vi "test_assignment.vi"() -> ()   [LabVIEW 2019]
panel:
  in  "OK Button":bool
  out "Indicator":bool
  out "x+y":dbl
  in  "tempInC":dbl(knob) scale=0.0..10.0
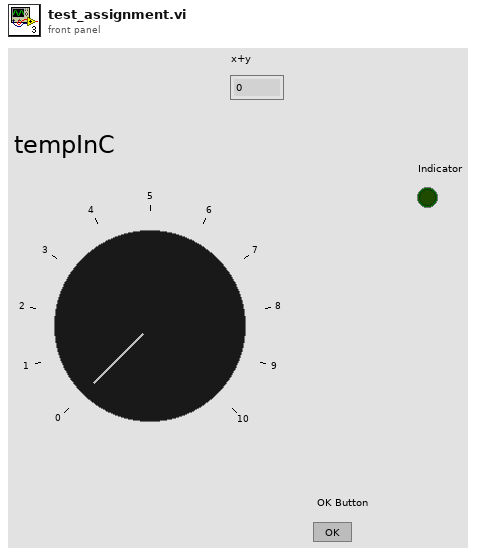
[diagram p1: front panel]
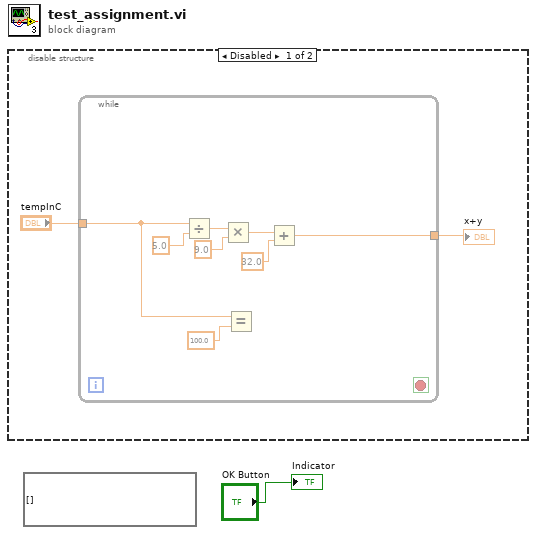
[diagram p0: block diagram]
diagram:
  (unwired) void[][][] []
  n1 = disable-structure shown="Disabled" {
    frame Disabled {
      n2 = while {
        tunnel: "tempInC" -> [w5]
        tunnel: [w6] -> w2
        stop <- _ stop-if-true
        n3 = Divide(x=w5, y=5.0) -> (x/y=w10:dbl)
        n4 = Multiply(x=w10, y=9.0) -> (x*y=w8:dbl)
        n5 = Equal?(x=w5, y=100.0) -> ()  [unwired: 1 out]
        n6 = Add(x=w8, y=32.0) -> (x+y=w6:dbl)
      }
      "x+y" <- w2
    }
    frame Enabled {
    }
  }
  "Indicator" <- "OK Button"
